vi "TxTestExample.vi"() -> ()   [LabVIEW 2015, in "QCA_DUT_Func.lvlib"]
uses:
  QCA_DUT_Func.lvlib
panel:
  out "return type 2":u8=1
  out "return type":u8
  in  "Cluster":T1={"numPackets"=0, "broadcast"=0, "flags"=28, "gainIdx"=0, "dacGain"=0, "paConfig"=0, "tpcm"=0, "txMode"=3, "channel"=5180, "rateBitIndex0"=97, "wlanMode"=8, "pktLen0"=1500, "txChain0"=0, "shortGuard"=0, "chanel2"=5290, "txpower0"=0.0, "antenna"=0, "bandwidth"=0}
  in  "Bin_file":string="D:\\4-Up-WLAN-Test-System\\board_data\\boardData_QCA9984_CUS239_5G_v1_001.bin"
  in  "chip_select":i32=3
  in  "DUT_IP":string="192.168.1.2"
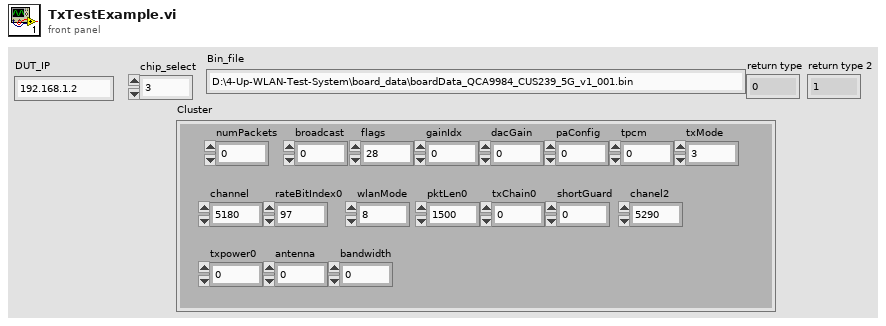
[diagram p1: front panel]
types:
  T1 = cluster{"numPackets":i32, "broadcast":i32, "flags":i32, "gainIdx":i32, "dacGain":i32, "paConfig":i32, "tpcm":i32, "txMode":i32, "channel":i32, "rateBitIndex0":i32, "wlanMode":i32, "pktLen0":i32, "txChain0":i32, "shortGuard":i32, "chanel2":i32, "txpower0":dbl, "antenna":i32, "bandwidth":i32}
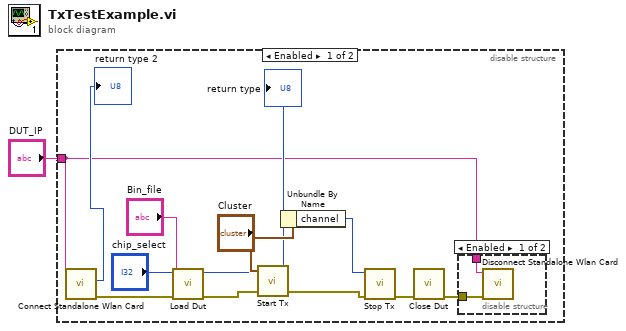
[diagram p0: block diagram]
diagram:
  n1 = disable-structure shown="Enabled" {
    disable-tunnel: "DUT_IP" -> [w2 _]
    frame Enabled {
      n2 = call "Connect Standalone Wlan Card.vi"("DUT_IP"=w2) -> ("error out"=w13:errorcluster, "return type"=→"return type 2":u8)  [unwired: 8 in, 1 out]
      n3 = call "Load Dut.vi"("error in (no error)"=w13, "Bin_file"="Bin_file", "chip_select"="chip_select") -> ("error out"=w8:errorcluster, "return type"=→"return type":u8)  [unwired: 6 in, 1 out]
      n4 = call "Start Tx.vi"("error in (no error)"=w8, "Cluster"="Cluster") -> ("error out"=w7:errorcluster)  [unwired: 3 in]
      n5 = Unbundle By Name("Cluster") -> ("channel"=w5:i32)
      n6 = call "Stop Tx.vi"("error in (no error)"=w7, "channel"=w5) -> ("error out"=w10:errorcluster)  [unwired: 8 in, 1 out]
      n7 = call "Close Dut.vi"("error in (no error)"=w10) -> ("error out"=w9:errorcluster)  [unwired: 10 in]
      n8 = disable-structure shown="Enabled" {
        disable-tunnel: w9 -> [w15 _]
        disable-tunnel: w2 -> [w14 _]
        frame Enabled {
          n9 = call "Disconnect Standalone Wlan Card.vi"("error in (no error)"=w15, "DUT_IP"=w14) -> ()  [unwired: 8 in, 2 out]
        }
        frame Disabled {
        }
      }
    }
    frame Disabled {
    }
  }
